vi "A Inches to Potentiometer.vi"(11 "Inches":dbl) -> (3 "Potentiometer":dbl)   [LabVIEW 2015]
uses:
  Robot Global Data.vi
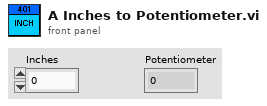
[diagram p1: front panel]
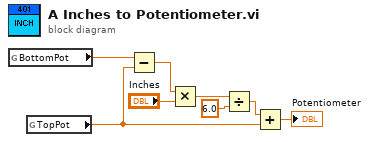
[diagram p0: block diagram]
diagram:
  n1 = global read "Robot Global Data.vi" "BottomPot"() -> (w2:dbl)
  n2 = global read "Robot Global Data.vi" "TopPot"() -> (w1:dbl)
  n3 = Subtract(x=w2, y=w1) -> (x-y=w8:dbl)
  n4 = Multiply(x=w8, y="Inches") -> (x*y=w6:dbl)
  n5 = Divide(x=w6, y=6.0) -> (x/y=w4:dbl)
  n6 = Add(x=w4, y=w1) -> (x+y=→"Potentiometer":dbl)
